vi "Read Key Names.vi"(8 "error in":errorcluster, 11 "Configuration in":refnum<class "Configuration.lvclass">) -> (0 "error out":errorcluster, 2 "Keys":string[](array[string]), 3 "Configuration out":refnum<class "Configuration.lvclass">)   [LabVIEW 2018, in "Configuration.lvlib" / "Configuration.lvclass"]
doc: "Read the keys stored in memory from the initialization."
uses:
  Configuration.lvclass
  Configuration.lvclass/Configuration.ctl
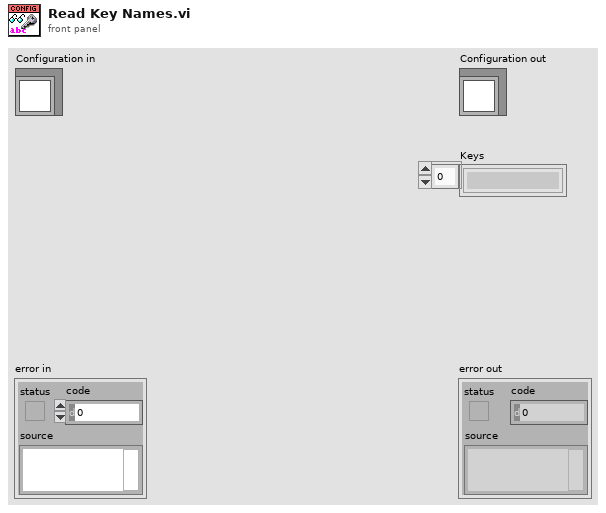
[diagram p1: front panel]
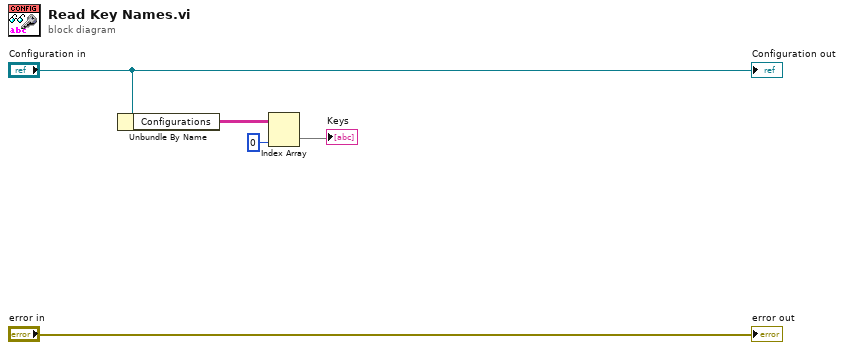
[diagram p0: block diagram]
diagram:
  n1 = Unbundle By Name("Configuration in") -> ("Configurations"=w3:string[][])
  n2 = Index Array(array=w3, index (col)=0 ("disabled index (col)")) -> (element=→"Keys":string[])  [unwired: 1 in]
  "error out" <- "error in"
  "Configuration out" <- "Configuration in"
